vi "Simple Serial.vi"() -> ()   [LabVIEW 2018]
doc: "This example performs a serial port write and a serial port read. The parameters set for the serial port must match the parameters of the connected instrument or device. The VISA Configure Serial Port VI sets the configuration parameters. The front panel displays the controls used to configure the basic parameters, such as baud rate, data bits, and parity. The VI passes the VISA resource name to other VIs that perform operations on that VISA resource. The VISA Write function sends a command to the serial device and the VISA Read function returns data based on the command. The VISA Close function then closes the reference to the serial device. It is important to close the reference; otherwise, further communication through that port might not be possible."
uses:
  Program Files (x86)/National Instruments/LabVIEW 2018/examples/Instrument IO/Serial/support/Serial - Settings.ctl
  <vilib>/Instr/_visa.llb/VISA Configure Serial Port (Instr).vi
panel:
  out "light intensity":u16
  out "red":u16
  out "green":u16
  out "blue":u16
  out "Button Sensor":bool
  out "Array 2":i32[](array[numeric])
  out "accX 2":i16
  out "accY 2":i16
  out "accZ 2":i16
  out "ultrasonic distance (mm)":dbl
  out "B4":bool
  out "B3":bool
  out "B2":bool
  out "B1":bool
  out "temperature":dbl
  out "accZ":i16
  out "accY":i16
  out "accX":i16
  out "batteryVoltage":dbl
  out "corruptedTicks":u8
  in  "Init":bool
  out "Array":string[](array[string])
  in  "Sync":bool
  in  "stop":bool
  in  "Serial Settings":T1={"baud rate"=9600, "data bits"=8, "parity"=enum."None", "stop bits"=10, "flow control"=0} {"flow control" items=["None"=0, "XON/XOFF"=1, "RTS/CTS"=2, "DTR/DSR"=4]; "stop bits" items=["1.0"=10, "1.5"=15, "2.0"=20]; "data bits" min=5 max=8 step=1; "baud rate" items=["75"=75, "110"=110, "134"=134, "150"=150, "300"=300, "600"=600, "1200"=1200, "1800"=1800, "2400"=2400, "4800"=4800, "7200"=7200, "9600"=9600, "14400"=14400, "19200"=19200, "28800"=28800, "38400"=38400, "56000"=56000, "57600"=57600, "115200"=115200, "128000"=128000, "230400"=230400]}
  out "bytes read":u32
  out "Response":string
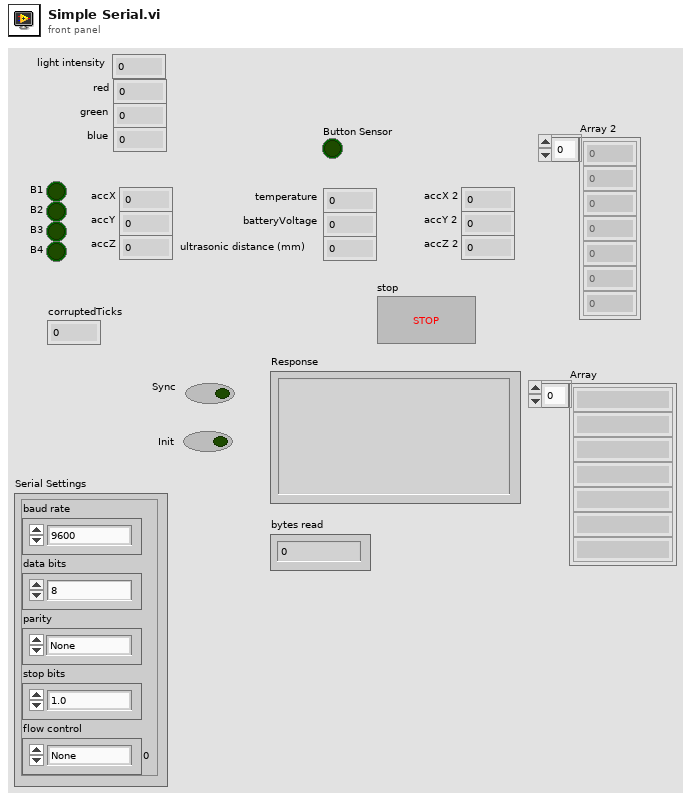
[diagram p1: front panel]
types:
  T1 = typedef "Serial - Settings.ctl" = cluster{"baud rate":u32, "data bits":u16, "parity":enum16{"None", "Odd", "Even", "Mark", "Space"}, "stop bits":u16, "flow control":u16}
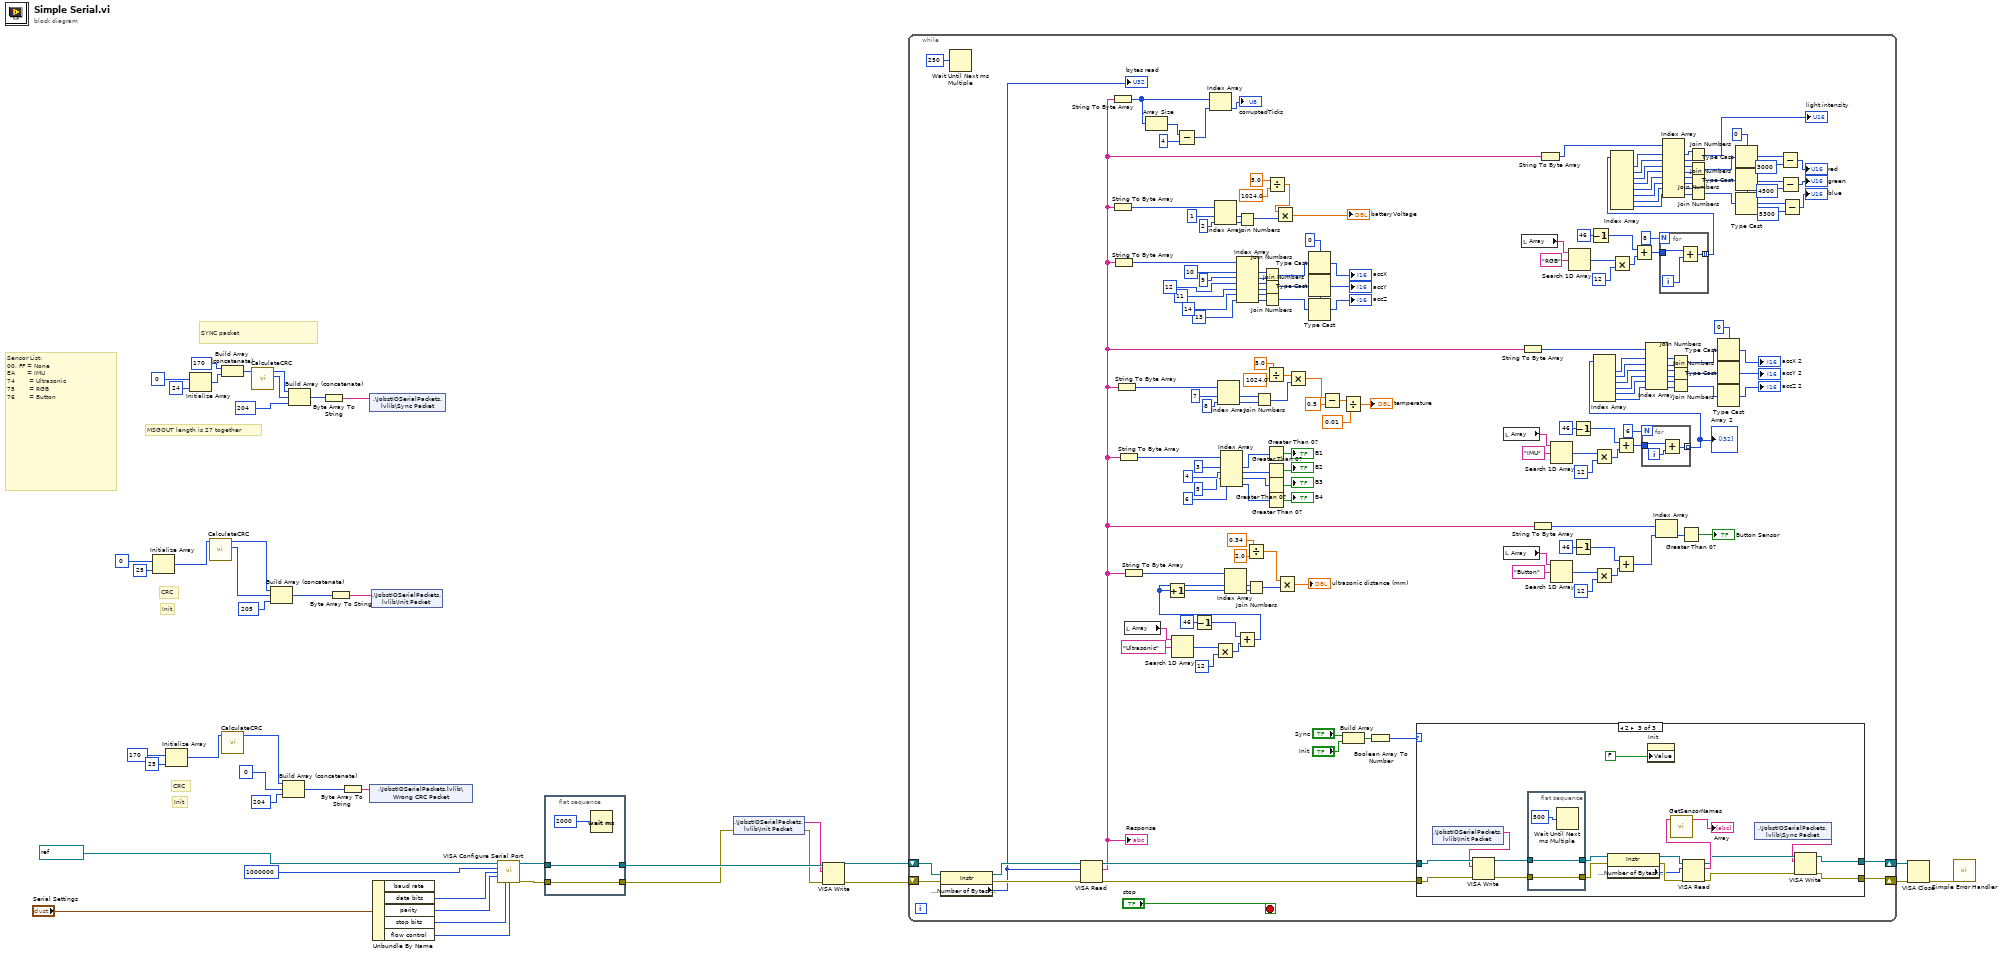
[diagram p0: block diagram]
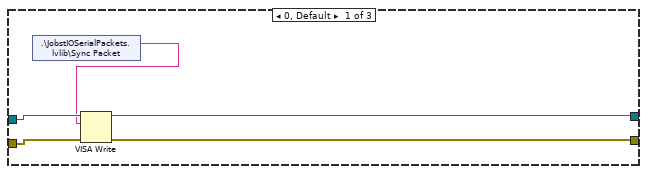
[diagram p2: hidden frame]
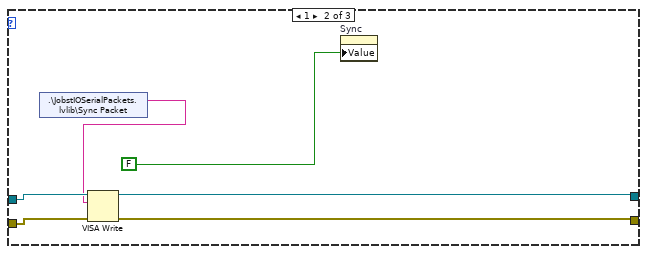
[diagram p3: hidden frame]
diagram:
  # "Init"
  # "CRC"
  # "Sensor List:\n00, FF = None\nEA      = IMU\n74       = Ultrasonic\n75       = RGB\n76       = Button"
  # "SYNC packet"
  # "Init"
  # "CRC"
  # "MSGOUT length is 27 together"
  n1 = Initialize Array(u8 0, 25 ("dimension size")) -> (w21:u8[])
  n2 = Initialize Array(u8 170, 25 ("dimension size")) -> (w17:u8[])
  n3 = Initialize Array(u8 0, 24 ("dimension size")) -> (w4:u8[])
  n4 = call "CalculateCRC.vi"("data in"=w21) -> ("CRC"=w19:u8, "data out"=w20:u8[])  [unwired: 9 in]
  n5 = Build Array (concatenate)(u8 170, w4) -> (w3:u8[])
  n6 = call "CalculateCRC.vi"("data in"=w17) -> ("data out"=w18:u8[])  [unwired: 9 in, 1 out]
  n7 = call "CalculateCRC.vi"("data in"=w3) -> ("CRC"=w1:u8, "data out"=w2:u8[])  [unwired: 9 in]
  n8 = Build Array (concatenate)(w20, w19, u8 205) -> (w30:u8[])
  n9 = Build Array (concatenate)(w18, u8 0, u8 204) -> (w15:u8[])
  n10 = Build Array (concatenate)(w2, w1, u8 204) -> (w22:u8[])
  n11 = Byte Array To String(unsigned byte array=w22) -> (string=w11:string)
  n12 = Byte Array To String(unsigned byte array=w30) -> (string=w10:string)
  n13 = Byte Array To String(unsigned byte array=w15) -> (string=w9:string)
  n14 = shared-variable ".\\JobstIOSerialPackets.lvlib\\Sync Packet"(w11) -> ()  [unwired: 1 in, 1 out]
  n15 = shared-variable ".\\JobstIOSerialPackets.lvlib\\Wrong CRC Packet"(w9) -> ()  [unwired: 1 in, 1 out]
  n16 = shared-variable ".\\JobstIOSerialPackets.lvlib\\Init Packet"(w10) -> ()  [unwired: 1 in, 1 out]
  n17 = Unbundle By Name("Serial Settings") -> ("data bits"=w37:u16, "parity"=w36:enum16{"None", "Odd", "Even", "Mark", "Space"}, "stop bits"=w35:u16, "flow control"=w34:u16)  [unwired: 1 out]
  n18 = call-poly "VISA Configure Serial Port"("VISA resource name"=refnum<visa-resource-name> "COM8", "baud rate (9600)"=u32 1000000, "data bits (8)"=w37, "parity (0:none)"=w36, "stop bits (10: 1 bit)"=w35, "flow control (0:none)"=w34) -> ("VISA resource name out"=w42:refnum<visa-resource-name>, "error out"=w43:errorcluster)  [unwired: 3 in, 5 out]
  n19 = flat-sequence {
    tunnel: w43 -> [w47]
    tunnel: [w47] -> w7
    tunnel: w42 -> [w46]
    tunnel: [w46] -> w26
    frame #0 {
      n20 = Wait (ms)(milliseconds to wait=u32 2000 ("delay before read (ms)")) -> ()  [unwired: 1 out]
    }
  }
  n21 = shared-variable ".\\JobstIOSerialPackets.lvlib\\Init Packet"(error in=w7) -> (w8:string, error out=w6:errorcluster)
  n22 = VISA Write(VISA resource name=w26, write buffer=w8, error in (no error)=w6) -> (VISA resource name out=w27:refnum<visa-resource-name>, error out=w28:errorcluster)  [unwired: 1 out]
  n23 = while {
    shift-right: [w211] -> w41
    shift-left: w28 -> [w224]
    shift-right: [w212] -> w40
    shift-left: w27 -> [w223]
    stop <- "stop" stop-if-true
    w73 = u16 0 ("index")
    w117 = i16 0 ("index")
    w186 = i16 0 ("index")
    n24 = property class="Instr"(reference=w223, error in=w224) -> (reference out=w222:refnum<visa-resource-name>, error out=w221:errorcluster, "Serial Settings:Number of Bytes at Serial Port"=w210:u32)
    "bytes read" <- w210
    n25 = Wait Until Next ms Multiple(millisecond multiple=u32 250) -> ()  [unwired: 1 out]
    n26 = VISA Read(VISA resource name=w222, byte count=w210, error in (no error)=w221) -> (VISA resource name out=w217:refnum<visa-resource-name>, read buffer=w62:string, error out=w218:errorcluster)  [unwired: 1 out]
    "Response" <- w62
    n27 = String To Byte Array(string=w62) -> (unsigned byte array=w205:u8[])
    n28 = String To Byte Array(string=w62) -> (unsigned byte array=w204:u8[])
    n29 = String To Byte Array(string=w62) -> (unsigned byte array=w197:u8[])
    n30 = String To Byte Array(string=w62) -> (unsigned byte array=w173:u8[])
    n31 = String To Byte Array(string=w62) -> (unsigned byte array=w165:u8[])
    n32 = String To Byte Array(string=w62) -> (unsigned byte array=w145:u8[])
    n33 = local read "Array"() -> (w147:string[])
    n34 = Array Size(array=w205) -> (size(s)=w209:i32)
    n35 = Search 1D Array(1D array=w147, element="Ultrasonic") -> (index of element=w142:i32)  [unwired: 1 in]
    n36 = Subtract(x=w209, y=4) -> (x-y=w207:i32)
    n37 = Decrement(x=46) -> (x-1=w140:i32)
    n38 = Index Array(array=w205, index=w207) -> (element=→"corruptedTicks":u8)
    n39 = Index Array(array=w204, index #1=1 ("index"), index #2=2 ("index")) -> (element #1=w201:u8, element #2=w200:u8)
    n40 = Multiply(x=w142, y=12) -> (x*y=w141:i32)
    n41 = Index Array(array=w173, index #1=7 ("index"), index #2=8 ("index")) -> (element #1=w176:u8, element #2=w177:u8)
    n42 = Index Array(array=w165, index #1=3 ("index"), index #2=4 ("index"), index #3=5 ("index"), index #4=6 ("index")) -> (element #1=w156:u8, element #2=w155:u8, element #3=w154:u8, element #4=w153:u8)
    n43 = Index Array(array=w197, index #1=10 ("index"), index #2=9 ("index"), index #3=12 ("index"), index #4=11 ("index"), index #5=14 ("index"), index #6=13 ("index")) -> (element #1=w192:u8, element #2=w191:u8, element #3=w190:u8, element #4=w189:u8, element #5=w188:u8, element #6=w187:u8)
    n44 = Add(x=w140, y=w141) -> (x+y=w139:i32)
    n45 = Increment(x=w139) -> (x+1=w138:i32)
    n46 = Index Array(array=w145, index #1=w139, index #2=w138) -> (element #1=w136:u8, element #2=w137:u8)
    n47 = Join Numbers(hi=w201, lo=w200) -> ((hi.lo)=w149:u16)
    n48 = Divide(x=0.34, y=2.0 ("x")) -> (x/y=w132:dbl)
    n49 = Join Numbers(hi=w136, lo=w137) -> ((hi.lo)=w133:u16)
    n50 = Join Numbers(hi=w176, lo=w177) -> ((hi.lo)=w167:u16)
    n51 = Join Numbers(hi=w192, lo=w191) -> ((hi.lo)=w182:u16)
    n52 = Join Numbers(hi=w189, lo=w190) -> ((hi.lo)=w181:u16)
    n53 = Join Numbers(hi=w187, lo=w188) -> ((hi.lo)=w180:u16)
    n54 = Divide(x=5.0, y=1024.0 ("x")) -> (x/y=w168:dbl)
    n55 = Greater Than 0?(x=w156) -> (x > 0?=→"B1":bool)
    n56 = Greater Than 0?(x=w155) -> (x > 0?=→"B2":bool)
    n57 = Greater Than 0?(x=w154) -> (x > 0?=→"B3":bool)
    n58 = Greater Than 0?(x=w153) -> (x > 0?=→"B4":bool)
    n59 = Divide(x=5.0 ("index"), y=1024.0 ("index")) -> (x/y=w150:dbl)
    n60 = Multiply(x=w150, y=w149) -> (x*y=→"batteryVoltage":dbl)
    n61 = Multiply(x=w132, y=w133) -> (x*y=→"ultrasonic distance (mm)":dbl)
    n62 = Multiply(x=w168, y=w167) -> (x*y=w166:dbl)
    n63 = Type Cast(type=w186, x=w182) -> (*(type *) &x=→"accX":i16)
    n64 = Type Cast(type=w186, x=w181) -> (*(type *) &x=→"accY":i16)
    n65 = Type Cast(type=w186, x=w180) -> (*(type *) &x=→"accZ":i16)
    n66 = Subtract(x=w166, y=0.5) -> (x-y=w171:dbl)
    n67 = Divide(x=w171, y=0.01) -> (x/y=→"temperature":dbl)
    n68 = Build Array("Sync", "Init") -> (w214:bool[])
    n69 = Boolean Array To Number(Boolean array=w214) -> (number=w213:u32)
    n70 = case shown="2" w213 {
      tunnel: w218 -> [w233 w240 w259]
      tunnel: w217 -> [w232 w239 w258]
      tunnel: [w235 w238 w243] -> w211
      tunnel: [w234 w237 w244] -> w212
      frame 0, Default {
        n71 = shared-variable ".\\JobstIOSerialPackets.lvlib\\Sync Packet"() -> (w231:string)  [unwired: 1 in, 1 out]
        n72 = VISA Write(VISA resource name=w232, write buffer=w231, error in (no error)=w233) -> (VISA resource name out=w234:refnum<visa-resource-name>, error out=w235:errorcluster)  [unwired: 1 out]
      }
      frame 1 {
        n73 = shared-variable ".\\JobstIOSerialPackets.lvlib\\Sync Packet"() -> (w236:string)  [unwired: 1 in, 1 out]
        n74 = VISA Write(VISA resource name=w239, write buffer=w236, error in (no error)=w240) -> (VISA resource name out=w237:refnum<visa-resource-name>, error out=w238:errorcluster)  [unwired: 1 out]
        n75 = property on="Sync" class="Bool (strict)"("Value"=FALSE ("Boolean")) -> ()  [unwired: 2 in, 2 out]
      }
      frame 2 {
        n76 = shared-variable ".\\JobstIOSerialPackets.lvlib\\Init Packet"() -> (w254:string)  [unwired: 1 in, 1 out]
        n77 = VISA Write(VISA resource name=w258, write buffer=w254, error in (no error)=w259) -> (VISA resource name out=w255:refnum<visa-resource-name>, error out=w256:errorcluster)  [unwired: 1 out]
        n78 = flat-sequence {
          tunnel: [w261] -> w252
          tunnel: w256 -> [w261]
          tunnel: [w260] -> w251
          tunnel: w255 -> [w260]
          frame #0 {
            n79 = Wait Until Next ms Multiple(millisecond multiple=u32 500) -> ()  [unwired: 1 out]
          }
        }
        n80 = property class="Instr"(reference=w251, error in=w252) -> (reference out=w248:refnum<visa-resource-name>, error out=w250:errorcluster, "Serial Settings:Number of Bytes at Serial Port"=w249:u32)
        n81 = property on="Init" class="Bool (strict)"("Value"=FALSE ("Init")) -> ()  [unwired: 2 in, 2 out]
        n82 = VISA Read(VISA resource name=w248, byte count=w249, error in (no error)=w250) -> (VISA resource name out=w245:refnum<visa-resource-name>, read buffer=w247:string, error out=w246:errorcluster)  [unwired: 1 out]
        n83 = call "GetSensorNames.vi"("read buffer"=w247) -> ("sensors names"=→"Array":string[])  [unwired: 10 in]
        n84 = shared-variable ".\\JobstIOSerialPackets.lvlib\\Sync Packet"() -> (w242:string)  [unwired: 1 in, 1 out]
        n85 = VISA Write(VISA resource name=w245, write buffer=w242, error in (no error)=w246) -> (VISA resource name out=w244:refnum<visa-resource-name>, error out=w243:errorcluster)  [unwired: 1 out]
      }
    }
    n86 = local read "Array"() -> (w110:string[])
    n87 = local read "Array"() -> (w100:string[])
    n88 = local read "Array"() -> (w80:string[])
    n89 = String To Byte Array(string=w62) -> (unsigned byte array=w118:u8[])
    n90 = String To Byte Array(string=w62) -> (unsigned byte array=w93:u8[])
    n91 = String To Byte Array(string=w62) -> (unsigned byte array=w72:u8[])
    n92 = Search 1D Array(1D array=w110, element="IMU") -> (index of element=w114:i32)  [unwired: 1 in]
    n93 = Search 1D Array(1D array=w100, element="Button") -> (index of element=w96:i32)  [unwired: 1 in]
    n94 = Search 1D Array(1D array=w80, element="RGB") -> (index of element=w76:i32)  [unwired: 1 in]
    n95 = Decrement(x=46) -> (x-1=w116:i32)
    n96 = Decrement(x=46) -> (x-1=w94:i32)
    n97 = Decrement(x=46) -> (x-1=w74:i32)
    n98 = Multiply(x=w114, y=12) -> (x*y=w115:i32)
    n99 = Multiply(x=w96, y=12) -> (x*y=w95:i32)
    n100 = Multiply(x=w76, y=12) -> (x*y=w75:i32)
    n101 = Add(x=w116, y=w115) -> (x+y=w109:i32)
    n102 = Add(x=w94, y=w95) -> (x+y=w92:i32)
    n103 = Add(x=w74, y=w75) -> (x+y=w81:i32)
    n104 = for {
      N: 6 -> [_]
      tunnel: w109 -> [w229]
      tunnel: [w228] -> w107 mode=indexing
      i -> [w230]
      n105 = Add(x=w229, y=w230) -> (x+y=w228:i32)
    }
    "Array 2" <- w107
    n106 = Index Array(array=w107) -> (element #1=w106:i32, element #2=w105:i32, element #3=w104:i32, element #4=w103:i32, element #5=w102:i32, element #6=w101:i32)  [unwired: 6 in]
    n107 = Index Array(array=w118, index #1=w106, index #2=w105, index #3=w104, index #4=w103, index #5=w102, index #6=w101) -> (element #1=w119:u8, element #2=w120:u8, element #3=w121:u8, element #4=w122:u8, element #5=w123:u8, element #6=w124:u8)
    n108 = Index Array(array=w93, index=w92) -> (element=w91:u8)
    n109 = for {
      N: 8 -> [_]
      tunnel: w81 -> [w227]
      tunnel: [w226] -> w83 mode=indexing
      i -> [w225]
      n110 = Add(x=w227, y=w225) -> (x+y=w226:i32)
    }
    n111 = Index Array(array=w83) -> (element #1=w51:i32, element #2=w52:i32, element #3=w84:i32, element #4=w85:i32, element #5=w86:i32, element #6=w87:i32, element #7=w88:i32, element #8=w89:i32)  [unwired: 8 in]
    n112 = Index Array(array=w72, index #1=w51, index #2=w52, index #3=w84, index #4=w85, index #5=w86, index #6=w87, index #7=w88, index #8=w89) -> (element #1=w49:u8, element #2=w50:u8, element #3=w71:u8, element #4=w70:u8, element #5=w69:u8, element #6=w68:u8, element #7=w67:u8, element #8=w66:u8)
    n113 = Join Numbers(hi=w119, lo=w120) -> ((hi.lo)=w128:u16)
    n114 = Join Numbers(hi=w122, lo=w121) -> ((hi.lo)=w129:u16)
    n115 = Join Numbers(hi=w124, lo=w123) -> ((hi.lo)=w130:u16)
    n116 = Greater Than 0?(x=w91) -> (x > 0?=→"Button Sensor":bool)
    n117 = Join Numbers(hi=w49, lo=w50) -> ((hi.lo)=→"light intensity":u16)
    n118 = Join Numbers(hi=w71, lo=w70) -> ((hi.lo)=w65:u16)
    n119 = Join Numbers(hi=w68, lo=w69) -> ((hi.lo)=w64:u16)
    n120 = Join Numbers(hi=w66, lo=w67) -> ((hi.lo)=w63:u16)
    n121 = Type Cast(type=w117, x=w128) -> (*(type *) &x=→"accX 2":i16)
    n122 = Type Cast(type=w117, x=w129) -> (*(type *) &x=→"accY 2":i16)
    n123 = Type Cast(type=w117, x=w130) -> (*(type *) &x=→"accZ 2":i16)
    n124 = Type Cast(type=w73, x=w65) -> (*(type *) &x=w61:u16)
    n125 = Type Cast(type=w73, x=w64) -> (*(type *) &x=w55:u16)
    n126 = Type Cast(type=w73, x=w63) -> (*(type *) &x=w54:u16)
    n127 = Subtract(x=w61, y=u16 3000) -> (x-y=→"red":u16)
    n128 = Subtract(x=w55, y=u16 4500) -> (x-y=→"green":u16)
    n129 = Subtract(x=w54, y=u16 5300) -> (x-y=→"blue":u16)
  }
  n130 = VISA Close(VISA resource name=w40, error in (no error)=w41) -> (error out=w39:errorcluster)
  n131 = call <vilib>:"Simple Error Handler.vi"("error in (no error)"=w39) -> ()  [unwired: 1 in, 8 out]
